vi "Main.vi"() -> ()   [LabVIEW 2020]
uses:
  support/Weather Data.ctl
  <vilib>/DAQmx/read.llb/DAQmx Read (Analog DBL 1Chan 1Samp).vi
  <vilib>/DAQmx/create/channels.llb/DAQmx Create Channel (AI-Temperature-Thermocouple).vi
  <vilib>/DAQmx/configure/timing.llb/DAQmx Timing (Sample Clock).vi
  <vilib>/DAQmx/miscellaneous.llb/DAQmx Fill In Error Info.vi
panel:
  out "Weather Data":T1
  out "Waveform Chart":dbl(graph)
  in  "Stop":bool
  in  "Lower Limit":dbl=20.0
  in  "Upper Limit":dbl=30.0
  in  "DAQmx Physical Channel":tag="PCI-6221/ai0"
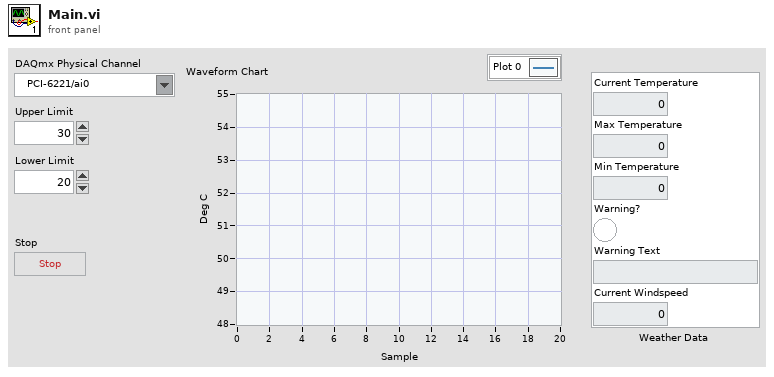
[diagram p1: front panel]
types:
  T1 = typedef "Weather Data.ctl" = cluster{"Current Temperature":dbl, "Max Temperature":dbl, "Min Temperature":dbl, "Warning?":bool, "Warning Text":string, "Current Windspeed":dbl}
  T2 = enum16{"open", "replace", "create", "open or create", "replace or create", "replace or create with confirmation"}
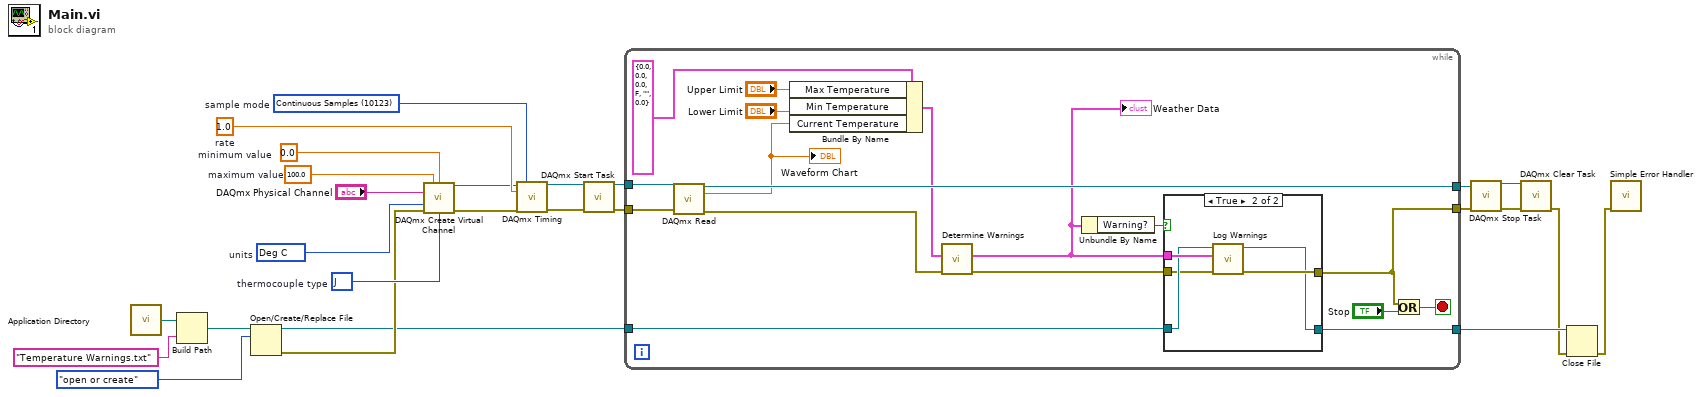
[diagram p0: block diagram]
diagram:
  w18 = 10123 items=["Finite Samples"=10178, "Continuous Samples"=10123, "Hardware Timed Single Point"=12522]  # sample mode
  w21 = 1.0  # rate
  w22 = 10072 items=["J"=10072, "K"=10073, "N"=10077, "R"=10082, "S"=10085, "T"=10086, "B"=10047, "E"=10055]  # thermocouple type
  w23 = 0.0  # minimum value
  w24 = 100.0  # maximum value
  w25 = 10143 items=["Deg C"=10143, "Deg F"=10144, "Kelvins"=10325, "Deg R"=10145, "From Custom Scale"=10065]  # units
  n1 = call <vilib>:"Application Directory.vi"() -> ("Application Directory"=w17:path)
  n2 = Build Path(base path=w17, name or relative path="Temperature Warnings.txt") -> (appended path=w15:path)
  n3 = Open/Create/Replace File(file path (use dialog)=w15, operation (0:open)=T2."open or create") -> (refnum out=w7:refnum<file>, error out=w13:errorcluster)  [unwired: 4 in, 1 out]
  n4 = call-poly <vilib>:"DAQmx Create Virtual Channel.vi"("maximum value"=w24, "minimum value"=w23, "physical channels"="DAQmx Physical Channel", "units"=w25, "error in"=w13, "thermocouple type"=w22) -> ("task out"=w20:refnum<k21>, "error out"=w19:errorcluster)  [unwired: 8 in]
  n5 = call-poly <vilib>:"DAQmx Timing.vi"("task/channels in"=w20, "sample mode"=w18, "rate"=w21, "error in"=w19) -> ("task out"=w12:refnum<k21>, "error out"=w11:errorcluster)  [unwired: 10 in]
  n6 = call <vilib>:"DAQmx Start Task.vi"("task/channels in"=w12, "error in"=w11) -> ("task out"=w10:refnum<k21>, "error out"=w9:errorcluster)  [unwired: 12 in]
  n7 = while {
    tunnel: w10 -> [w43]
    tunnel: w9 -> [w42]
    tunnel: [w39] -> w8
    tunnel: w7 -> [w36]
    tunnel: [w35] -> w3
    tunnel: [w34] -> w6
    stop <- w33 stop-if-true
    n8 = call-poly <vilib>:"DAQmx Read.vi"("task/channels in"=w43, "error in"=w42) -> ("task out"=w39:refnum<k21>, "data"=w27:dbl, "error out"=w37:errorcluster)  [unwired: 11 in]
    "Waveform Chart" <- w27
    n9 = Bundle By Name(cluster=T1 {"Current Temperature"=0.0, "Max Temperature"=0.0, "Min Temperature"=0.0, "Warning?"=FALSE, "Warning Text"="", "Current Windspeed"=0.0} ("Weather Data"), "Max Temperature"="Upper Limit", "Min Temperature"="Lower Limit", "Current Temperature"=w27) -> (w38:T1)
    n10 = call "Determine Warnings.vi"("Error In"=w37, "Weather Data In"=w38) -> ("Error Out"=w30:errorcluster, "Weather Data Out"=w28:T1)  [unwired: 8 in]
    "Weather Data" <- w28
    n11 = Unbundle By Name(w28) -> ("Warning?"=w31:bool)
    n12 = case shown="True" w31 {
      tunnel: w36 -> [w45 w48]
      tunnel: w28 -> [_ w50]
      tunnel: [w44 w49] -> w34
      tunnel: [w45 w47] -> w35
      tunnel: w30 -> [w44 w46]
      frame False {
      }
      frame True {
        n13 = call "Log Warnings.vi"("Error In"=w46, "Weather Data"=w50, "file ref in"=w48) -> ("Error Out"=w49:errorcluster, "file ref out"=w47:refnum<file>)  [unwired: 7 in]
      }
    }
    n14 = Or(x=w34, y="Stop") -> (x .or. y?=w33:bool)
  }
  n15 = call <vilib>:"DAQmx Stop Task.vi"("task/channels in"=w8, "error in"=w6) -> ("task out"=w5:refnum<k21>, "error out"=w4:errorcluster)  [unwired: 12 in]
  n16 = call <vilib>:"DAQmx Clear Task.vi"("task in"=w5, "error in"=w4) -> ("error out"=w2:errorcluster)  [unwired: 13 in]
  n17 = Close File(refnum=w3, error in=w2) -> (error out=w1:errorcluster)  [unwired: 1 out]
  n18 = call <vilib>:"Simple Error Handler.vi"("error in (no error)"=w1) -> ()  [unwired: 4 in, 5 out]
